vi "Machine Inspect [FPGA]C.vi"() -> ()   [LabVIEW 2016]
uses:
  <vilib>/Platform/TimedLoop/XDataNode/timing_clust.ctl
  <vilib>/Platform/TimedLoop/XDataNode/nitl_modes.ctl
  <vilib>/Platform/TimedLoop/XDataNode/wakeup.ctl
  <vilib>/rvi/Emulation/niFpgaGetClockAttributes.vi
  <vilib>/rvi/Emulation/niFpgaSctlEmulationGetInTimedLoop.vi
  <vilib>/rvi/Emulation/niFpgaEmulationReportErrorSimple.vi
  <vilib>/rvi/Emulation/niFpgaProcessEmulError.vi
  <vilib>/rvi/interface/RandomDataEmulation/niFpgaRandomDataHandleErrors.vi
  <vilib>/rvi/eio/common/nirviEmuTemplateMethod_errors.vi
  <vilib>/rvi/Emulation/niFpgaCriticalErrorInLSC.vi
  <vilib>/rvi/DataTransferAndStorage/Container/XNode/niFpgaContainer.xnode
  <vilib>/rvi/interface/RandomDataEmulation/nirviRandomDataFpgaReadWriteTemplate.vi
  <vilib>/eio/EIONode/EIONode.xnode
  <vilib>/Platform/TimedLoop/XDataNode/XDataNode.xnode
  <vilib>/Platform/TimedLoop/XDataNode/XDNodeRunTimeDep.lvlib
panel:
  in  "Gain":u32
  out "E-Stop":bool
  in  "PWM":bool
  out "Position":i16
  in  "Reset":bool
  # "Encoder Loop"
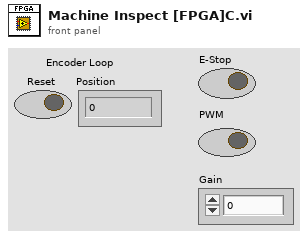
[diagram p1: front panel]
types:
  T1 = typedef "XDNodeRunTimeDep.lvlib/timing_clust.ctl" = cluster{"Expected End [f-1]":u64, "Actual End [f-1]":u64, "Finished Late? [f-1]":bool, "Expected End [i-1]":u64, "Actual End [i-1]":u64, "Finished Late? [i-1]":bool, "Expected Start [i]":u64, "Actual Start [i]":u64, "Expected Start [f]":u64, "Actual Start [f]":u64, "Source Name":string, "Structure Name":string, "Period":i64, "Deadline":i64, "Offset":i64, "Start":i64, "Priority":i32, "Timeout":i32, "Mode":T2, "Wakeup Reason":T3, "Error":errorcluster, "Source Type":string, "Secondary Source Type":string, "Global End Time":u64, "Global Start Time":u64, "Frame Duration":u64, "Iteration Duration":u64, "Assigned CPU":i32, "I/O Scan Engine Mode":u32}
  T2 = typedef "XDNodeRunTimeDep.lvlib/nitl_modes.ctl" = enum32{"No Change", "Process missed periods, maintain original phase", "Discard missed periods, maintain original phase", "Process missed periods, ignore original phase", "Discard missed periods, ignore original phase"}
  T3 = typedef "XDNodeRunTimeDep.lvlib/wakeup.ctl" = enum32{"Normal", "Aborted", "Asynchronous wakeup", "Timing source error", "Timed loop error", "Timeout"}
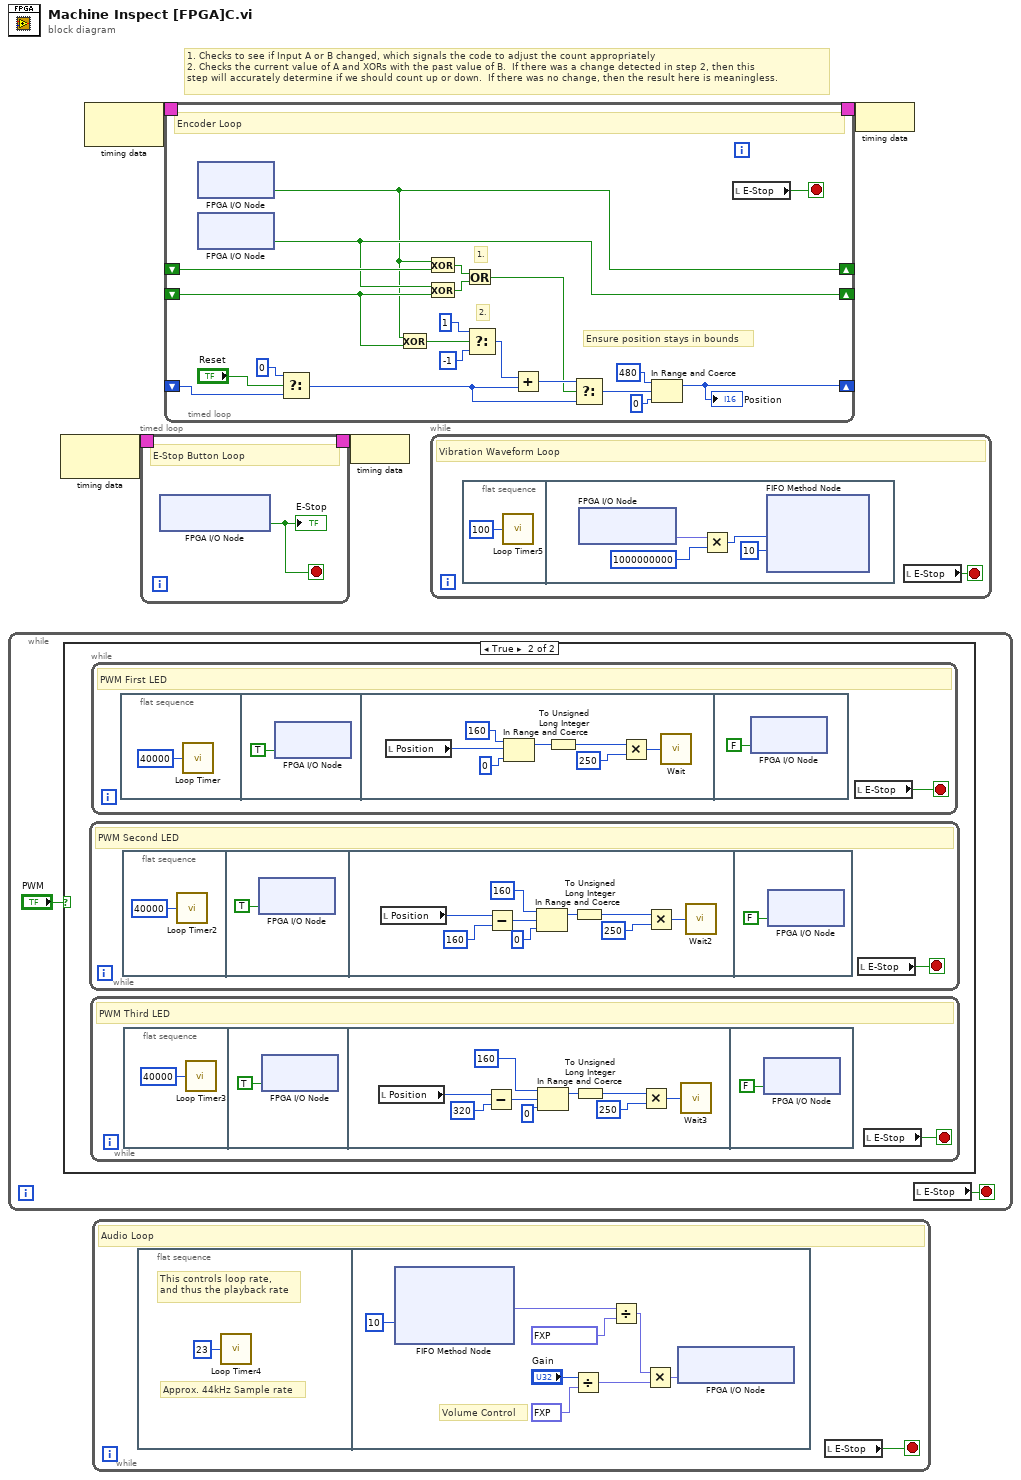
[diagram p0: block diagram]
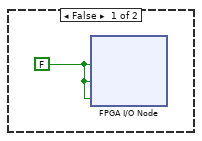
[diagram p2: hidden frame]
diagram:
  # "1. Checks to see if Input A or B changed, which signals the code to adjust the count appropriately\n2. Checks the current value of A and XORs with the past value of B.  If there was a change detected in step 2, then this \nstep will accurately determine if we should count up or down.  If there was no change, then the result here is meaningless."
  n1 = while {
    stop <- w5 stop-if-true
    n2 = case shown="True" "PWM" {
      frame False {
        w7 = FALSE ("DIO4")
        n3 = xnode "FPGA I/O Node"("LED1"=w7, "LED2"=w7, "LED3"=w7) -> ()  [unwired: 3 in, 3 out]
      }
      frame True {
        n4 = while {
          stop <- w21 stop-if-true
          # "PWM Second LED"
          n5 = flat-sequence {
            frame #0 {
              n6 = call "Loop Timer2"("Count(Ticks)"=u32 40000) -> ()  [unwired: 1 out]
            }
            frame #1 {
              n7 = xnode "FPGA I/O Node"("LED2"=TRUE ("DIO5")) -> ()  [unwired: 1 in, 1 out]
            }
            frame #2 {
              n8 = local read "Position"() -> (w26:i16)
              n9 = Subtract(x=w26, y=i16 160) -> (x-y=w28:i16)
              n10 = In Range and Coerce(upper limit=i16 160, x=w28, lower limit=i16 0) -> (coerced(x)=w25:i16)  [unwired: 1 out]
              n11 = To Unsigned Long Integer(number=w25) -> (unsigned 32bit integer=w24:u32)
              n12 = Multiply(x=w24, y=u32 250) -> (x*y=w29:u32)
              n13 = call "Wait2"("Count(Ticks)"=w29) -> ()  [unwired: 1 out]
            }
            frame #3 {
              n14 = xnode "FPGA I/O Node"("LED2"=FALSE ("DIO5")) -> ()  [unwired: 1 in, 1 out]
            }
          }
          n15 = local read "E-Stop"() -> (w21:bool)
        }
        n16 = while {
          stop <- w8 stop-if-true
          # "PWM Third LED"
          n17 = flat-sequence {
            frame #0 {
              n18 = call "Loop Timer3"("Count(Ticks)"=u32 40000) -> ()  [unwired: 1 out]
            }
            frame #1 {
              n19 = xnode "FPGA I/O Node"("LED3"=TRUE ("DIO5")) -> ()  [unwired: 1 in, 1 out]
            }
            frame #2 {
              n20 = local read "Position"() -> (w13:i16)
              n21 = Subtract(x=w13, y=i16 320) -> (x-y=w14:i16)
              n22 = In Range and Coerce(upper limit=i16 160, x=w14, lower limit=i16 0) -> (coerced(x)=w12:i16)  [unwired: 1 out]
              n23 = To Unsigned Long Integer(number=w12) -> (unsigned 32bit integer=w11:u32)
              n24 = Multiply(x=w11, y=u32 250) -> (x*y=w16:u32)
              n25 = call "Wait3"("Count(Ticks)"=w16) -> ()  [unwired: 1 out]
            }
            frame #3 {
              n26 = xnode "FPGA I/O Node"("LED3"=FALSE ("DIO5")) -> ()  [unwired: 1 in, 1 out]
            }
          }
          n27 = local read "E-Stop"() -> (w8:bool)
        }
        n28 = while {
          stop <- w34 stop-if-true
          # "PWM First LED"
          n29 = flat-sequence {
            frame #0 {
              n30 = call "Loop Timer"("Count(Ticks)"=u32 40000) -> ()  [unwired: 1 out]
            }
            frame #1 {
              n31 = xnode "FPGA I/O Node"("LED1"=TRUE ("DIO5")) -> ()  [unwired: 1 in, 1 out]
            }
            frame #2 {
              n32 = local read "Position"() -> (w39:i16)
              n33 = In Range and Coerce(upper limit=i16 160, x=w39, lower limit=i16 0) -> (coerced(x)=w38:i16)  [unwired: 1 out]
              n34 = To Unsigned Long Integer(number=w38) -> (unsigned 32bit integer=w37:u32)
              n35 = Multiply(x=w37, y=u32 250) -> (x*y=w40:u32)
              n36 = call "Wait"("Count(Ticks)"=w40) -> ()  [unwired: 1 out]
            }
            frame #3 {
              n37 = xnode "FPGA I/O Node"("LED1"=FALSE ("DIO5")) -> ()  [unwired: 1 in, 1 out]
            }
          }
          n38 = local read "E-Stop"() -> (w34:bool)
        }
      }
    }
    n39 = local read "E-Stop"() -> (w5:bool)
  }
  n40 = node-c288() -> (w2:T1)  [unwired: 1 in]
  n41 = node-c288() -> (w4:T1)  [unwired: 1 in]
  n42 = while {
    stop <- w45 stop-if-true
    # "Audio Loop"
    n43 = flat-sequence {
      frame #0 {
        # "Approx. 44kHz Sample rate"
        # "This controls loop rate,\nand thus the playback rate"
        n44 = call "Loop Timer4"("Count(uSec)"=u32 23) -> ()  [unwired: 1 out]
      }
      frame #1 {
        # "Volume Control"
        n45 = xnode ("FIFO Method Node")("Timeout"=10) -> ("Element"=w50:fxp<+/-,32,16>)  [unwired: 1 in, 2 out]
        n46 = Divide(x="Gain", y=fxp<+/-,32,16> 1000.0 ("Gain")) -> (x/y=w51:fxp<+/-,32,16>)
        n47 = Divide(x=w50, y=fxp<+/-,64,36> 1000000000.0 ("x*y")) -> (x/y=w48:fxp<+/-,64,34>)
        n48 = Multiply(x=w48, y=w51) -> (x*y=w47:fxp<+/-,64,50>)
        n49 = xnode "FPGA I/O Node"("Audio Output"=w47) -> ()  [unwired: 1 in, 1 out]
      }
    }
    n50 = local read "E-Stop"() -> (w45:bool)
  }
  n51 = timed-loop {
    timing: w2 -> [_]
    timing-out: [_] -> w1
    stop <- w55 stop-if-true
    # "E-Stop Button Loop"
    n52 = xnode "FPGA I/O Node"() -> ("Right Button"=w55:bool)  [unwired: 1 in, 1 out]
    "E-Stop" <- w55
  }
  n53 = timed-loop {
    shift-left: _ -> [w66]
    shift-right: [w65] -> _
    shift-left: _ -> [w75]
    shift-right: [w63] -> _
    shift-left: _ -> [w71]
    shift-right: [w58] -> _
    timing: w4 -> [_]
    timing-out: [_] -> w3
    stop <- w59 stop-if-true
    # "2."
    # "1."
    # "Ensure position stays in bounds"
    # "Encoder Loop"
    n54 = xnode "FPGA I/O Node"() -> ("DIO10"=w58:bool)  [unwired: 1 in, 1 out]
    n55 = xnode "FPGA I/O Node"() -> ("DIO11"=w65:bool)  [unwired: 1 in, 1 out]
    n56 = Select(t=i16 0, s="Reset", f=w75) -> (s? t:f=w76:i16)
    n57 = Exclusive Or(1:w66, 2:w58) -> (0:w67:bool)
    n58 = Exclusive Or(1:w71, 2:w58) -> (0:w69:bool)
    n59 = Exclusive Or(1:w66, 2:w65) -> (0:w70:bool)
    n60 = Or(x=w69, y=w70) -> (x .or. y?=w68:bool)
    n61 = Select(t=i16 1, s=w67, f=i16 -1) -> (s? t:f=w74:i16)
    n62 = Add(x=w74, y=w76) -> (x+y=w78:i16)
    n63 = Select(t=w78, s=w68, f=w76) -> (s? t:f=w64:i16)
    n64 = In Range and Coerce(upper limit=i16 480, x=w64, lower limit=i16 0) -> (coerced(x)=w63:i16)  [unwired: 1 out]
    "Position" <- w63
    n65 = local read "E-Stop"() -> (w59:bool)
  }
  n66 = node-c288(w1) -> ()
  n67 = while {
    stop <- w81 stop-if-true
    # "Vibration Waveform Loop"
    n68 = flat-sequence {
      frame #0 {
        n69 = call "Loop Timer5"("Count(uSec)"=u32 100) -> ()  [unwired: 1 out]
      }
      frame #1 {
        n70 = xnode "FPGA I/O Node"() -> ("Sine Wave"=w85:fxp<+/-,24,5>)  [unwired: 1 in, 1 out]
        n71 = Multiply(x=w85, y=1000000000) -> (x*y=w83:i32)
        n72 = xnode ("FIFO Method Node")("Element"=w83, "Timeout"=10) -> ()  [unwired: 1 in, 2 out]
      }
    }
    n73 = local read "E-Stop"() -> (w81:bool)
  }
  n74 = node-c288(w3) -> ()
